vi "MainUI.vi"() -> ()   [LabVIEW 2020]
uses:
  <vilib>/Utility/file.llb/Write Delimited Spreadsheet (string).vi
panel:
  in  "Save flattened data (memory hungry)":bool
  in  "Polarity":T1={"auto detect"=TRUE, "Polarity"=enum."falling"}
  in  "Measurement info":T2={"Det index"=0, "Clk index"=1, "Avg range"=1e-08}
  out "System Waveform Graph":cluster{"t0":dbl, "dt":dbl, "Y":dbl[]}[](graph) caption="ST Screen 3778 w02 no pull 32 - Beam reg23 Setting 7F-7E-7F-7F"
  in  "File extension":string="txt"
  out "Waveform Graph rise":cluster{"t0":dbl, "dt":dbl, "Y":dbl[]}[](graph)
  out "Waveform Graph fall":cluster{"t0":dbl, "dt":dbl, "Y":dbl[]}[](graph)
  out "data":string[](array[string])
  in  "File Path":path
  in  "Save extracted numbers":bool=TRUE
  in  "Filename has to include:":string
  in  "Play":bool
  in  "Exit":bool
  out "Heading":string[](array[string])=["reg23", "State", "Initial", "State", "Final"]
  out "Progress Bar":u8(slide) scale=0.0..100.0
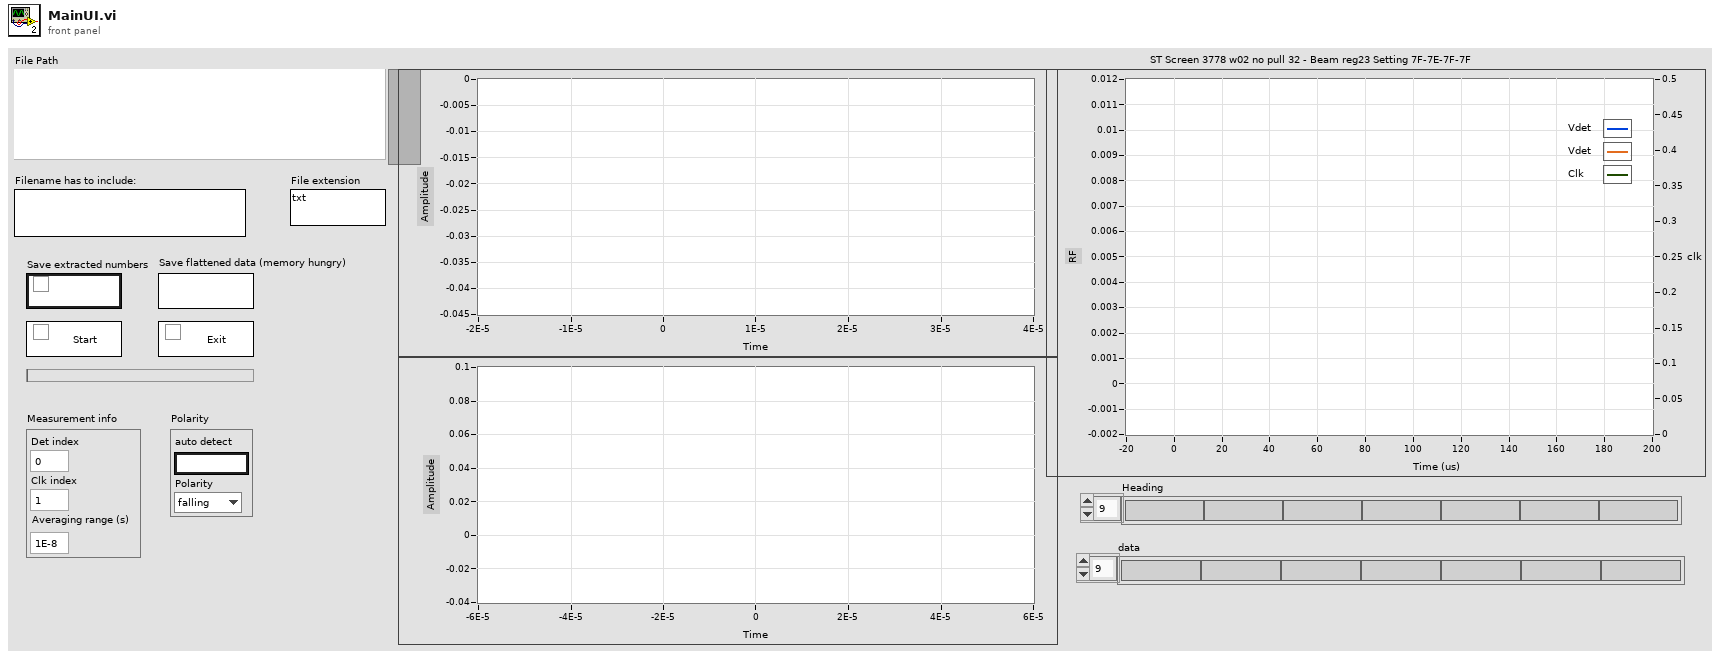
[diagram p1: front panel]
types:
  T1 = cluster{"auto detect":bool, "Polarity":enum16{"falling", "rising"}}
  T2 = cluster{"Det index":i32, "Clk index":i32, "Avg range":dbl}
  T3 = enum8{"Enabled", "Disabled", "Disabled and Grayed Out"}
  T4 = typedef "Timing measurements.ctl" = cluster{"Polarity":enum16{"falling", "rising"}, "low state level":dbl, "high state level":dbl, "t0 (us)":dbl, "Transition duration 10% (us)":dbl, "pre-undershoot 10% (%)":dbl, "pre-overshoot 10% (%)":dbl, "post-undershoot 10% (%)":dbl, "post-overshoot 10% (%)":dbl, "measurement info 10%":cluster{"start time":dbl, "end time":dbl, "ref levels":cluster{"high ref level":dbl, "mid ref level":dbl, "low ref level":dbl, "ref units":u16}}, "Settling time 5% (us)":dbl, "pre-undershoot 5% (%)":dbl, "pre-overshoot 5% (%)":dbl, "post-undershoot 5% (%)":dbl, "post-overshoot 5% (%)":dbl, "measurement info 5%":cluster{"start time":dbl, "end time":dbl, "ref levels":cluster{"high ref level":dbl, "mid ref level":dbl, "low ref level":dbl, "ref units":u16}}, "t0 to 5% (us)":dbl, "t0 to 10% (us)":dbl, "sclk edge":i32}
  T5 = cluster{"start time":dbl, "end time":dbl, "ref levels":cluster{"high ref level":dbl, "mid ref level":dbl, "low ref level":dbl, "ref units":u16}}
  T6 = cluster{"high ref level":dbl, "mid ref level":dbl, "low ref level":dbl, "ref units":u16}
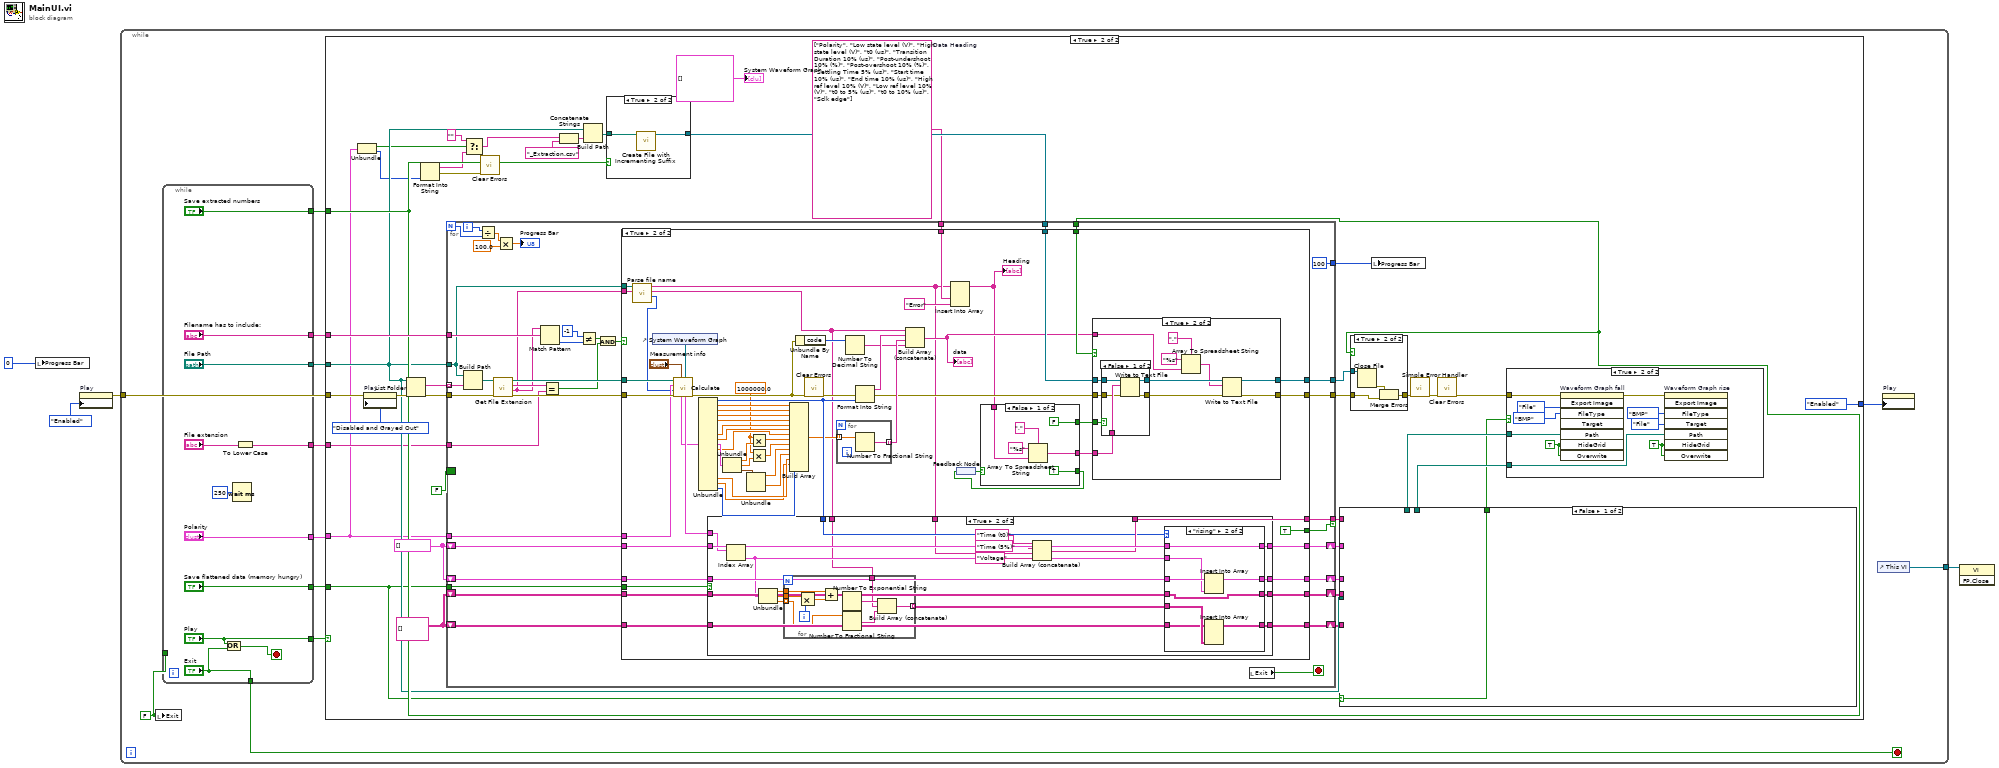
[diagram p0: block diagram]
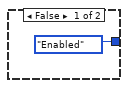
[diagram p2: hidden frame]
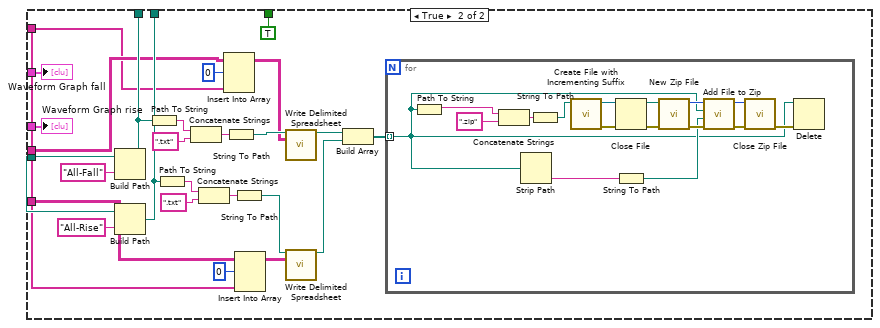
[diagram p4: hidden frame]
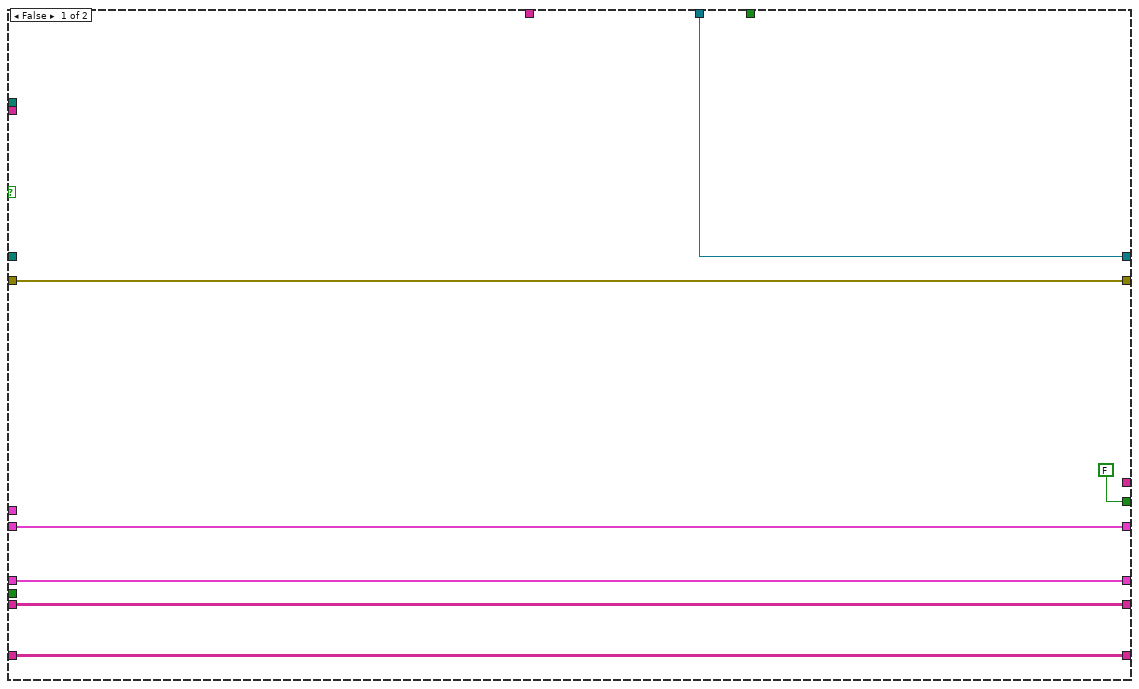
[diagram p7: hidden frame]
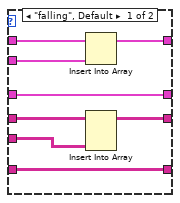
[diagram p9: hidden frame]
diagram:
  n1 = local write "Progress Bar"(u8 0 ("Horizontal Progress Bar")) -> ()
  n2 = property on="Play" class="Bool"("DisabledEnum"=T3."Enabled" ("Disabled")) -> (error out=w2:errorcluster)  [unwired: 2 in, 1 out]
  n3 = while {
    tunnel: w2 -> [w11]
    tunnel: [w8] -> w1
    stop <- w12 stop-if-true
    w10 = FALSE ("Exit")
    n4 = local write "Exit"(w10) -> ()
    n5 = while {
      tunnel: ["File Path"] -> w16
      tunnel: ["Filename has to include:"] -> w15
      tunnel: ["Save extracted numbers"] -> w14
      tunnel: ["Play"] -> w13
      tunnel: ["Exit"] -> w12
      tunnel: w10 -> [_]
      tunnel: [w311] -> w9
      tunnel: ["Polarity"] -> w7
      tunnel: ["Save flattened data (memory hungry)"] -> w5
      stop <- w315 stop-if-true
      n6 = Or(x="Play", y="Exit") -> (x .or. y?=w315:bool)
      n7 = Wait (ms)(milliseconds to wait=u32 250) -> ()  [unwired: 1 out]
      n8 = To Lower Case(string="File extension") -> (all lower case string=w311:string)
    }
    n9 = case shown="True" w13 {
      tunnel: w16 -> [_ w45]
      tunnel: w15 -> [_ w56]
      tunnel: w14 -> [_ w54]
      tunnel: w11 -> [_ w46]
      tunnel: w9 -> [_ w32]
      tunnel: w7 -> [_ w24]
      tunnel: [T3."Enabled" ("Disabled") T3."Enabled" ("Disabled")] -> w6
      tunnel: w5 -> [_ w28]
      frame False {
      }
      frame True {
        w35 = string[] ["Polarity", "Low state level (V)", "High state level (V)", "t0 (us)", "Transition Duration 10% (us)", "Post-undershoot 10% (%)", "Post-overshoot 10% (%)", "Settling Time 5% (us)", "Start time 10% (us)", "End time 10% (us)", "High ref level 10% (V)", "Low ref level 10% (V)", "t0 to 5% (us)", "t0 to 10% (us)", "Sclk edge"]  # Data Heading
        w39 = string[][] []
        w41 = cluster{"t0":dbl, "dt":dbl, "Y":dbl[]}[] []
        n10 = Unbundle(w24) -> ("auto detect"=w23:bool, "Polarity"=w21:enum16{"falling", "rising"})
        n11 = property on="Play" class="Bool"(error in=w46, "DisabledEnum"=T3."Disabled and Grayed Out" ("Disabled")) -> (error out=w48:errorcluster)  [unwired: 1 in, 1 out]
        n12 = List Folder(path=w45, error in=w48) -> (filenames=w58:string[], error out=w57:errorcluster)  [unwired: 2 in, 2 out]
        n13 = Format Into String(w21) -> (resulting string=w20:string, error out=w18:errorcluster)  [unwired: 3 in]
        n14 = Select(t="", s=w23, f=w20) -> (s? t:f=w22:string)
        n15 = call <vilib>:"Clear Errors.vi"("error in (no error)"=w18) -> ()  [unwired: 5 in, 2 out]
        n16 = Concatenate Strings(w22, "_Extraction.csv" ("string")) -> (w25:string)
        n17 = Build Path(base path=w45, name or relative path=w25) -> (appended path=w55:path)
        n18 = case shown="True" w54 {
          tunnel: w55 -> [_ w118]
          tunnel: [_ w117] -> w53
          frame False {
          }
          frame True {
            n19 = call <vilib>:"Create File with Incrementing Suffix.vi"("file path"=w118) -> ("refnum out"=w117:refnum<file>)  [unwired: 8 in, 2 out]
          }
        }
        n20 = for {
          N -> [w146]
          tunnel: w45 -> [w119]
          tunnel: w57 -> [w156]
          tunnel: w58 -> [w123] mode=indexing
          tunnel: w56 -> [w151]
          tunnel: w54 -> [w150]
          tunnel: w53 -> [w149]
          tunnel: [w148] -> w52
          border: FALSE -> [_]
          tunnel: [u8 100 ("Horizontal Progress Bar")] -> w50
          shift-right: [w140] -> w40
          shift-left: w41 -> [w139]
          shift-right: [w137] -> w44
          shift-left: w41 -> [w138]
          shift-right: [w136] -> w38
          shift-left: w39 -> [w134]
          shift-right: [w135] -> w36
          shift-left: w39 -> [w133]
          tunnel: [w132] -> w37 if=w131
          tunnel: w35 -> [w130]
          tunnel: [w129] -> w34
          tunnel: w32 -> [w124]
          tunnel: w24 -> [w122]
          tunnel: w28 -> [w121]
          i -> [w147]
          stop <- w141 stop-if-true
          n21 = Build Path(base path=w119, name or relative path=w123) -> (appended path=w154:path)
          n22 = Divide(x=w147, y=w146) -> (x/y=w145:dbl)
          n23 = call <vilib>:"Get File Extension.vi"("error in (no error)"=w156, "file"=w154) -> ("error out"=w155:errorcluster, "filename without extension"=w120:string, "lowercase file extension"=w126:string, "dup file"=w152:path)  [unwired: 5 in, 1 out]
          n24 = Multiply(x=w145, y=100.0) -> (x*y=→"Progress Bar":dbl)
          n25 = Match Pattern(string=w120, regular expression=w151) -> (offset past match=w153:i32)  [unwired: 1 in, 3 out]
          n26 = Equal?(x=w126, y=w124) -> (x = y?=w125:bool)
          n27 = Not Equal?(x=-1, y=w153) -> (x != y?=w128:bool)
          n28 = And(x=w128, y=w125) -> (x .and. y?=w127:bool)
          n29 = case shown="True" w127 {
            tunnel: w152 -> [_ w218]
            tunnel: [w163 w227] -> w129
            tunnel: w155 -> [w163 w219]
            tunnel: w150 -> [_ w226]
            tunnel: w149 -> [w164 w223]
            tunnel: [w164 w222] -> w148
            tunnel: [w162 w212] -> w140
            tunnel: w139 -> [w162 w213]
            tunnel: w138 -> [w161 w211]
            tunnel: [w161 w210] -> w137
            tunnel: [w159 w209] -> w136
            tunnel: [w160 w208] -> w135
            tunnel: w134 -> [w159 w207]
            tunnel: w133 -> [w160 w206]
            tunnel: [_ w204] -> w132
            tunnel: [FALSE TRUE] -> w131
            tunnel: w130 -> [_ w201]
            tunnel: w122 -> [_ w173]
            tunnel: w121 -> [_ w169]
            tunnel: w120 -> [_ w168]
            tunnel: w119 -> [_ w167]
            frame False {
            }
            frame True {
              w170 = 1000000.0 ("y")
              n30 = call "Parse file name.vi"("filename without extension"=w168, "File Path"=w167) -> ("Changed reg"=w172:u8, "Part info"=w166:string[], "Part info Header"=w165:string[])  [unwired: 7 in]
              n31 = control-ref of="System Waveform Graph"() -> (w180:refnum<vi>)
              n32 = call "Calculate.vi"("WFGraph Refnum"=w180, "Measurement info"="Measurement info", "error in"=w219, "Changed reg"=w172, "Polarity"=w173, "file (use dialog)"=w218) -> ("error out"=w176:errorcluster, "Waveform data out"=w198:cluster{"t0":dbl, "dt":dbl, "Y":dbl[]}[], "Timing measurements"=w197:T4)  [unwired: 1 in, 2 out]
              n33 = Unbundle(w197) -> ("Polarity"=w203:enum16{"falling", "rising"}, "low state level"=w195:dbl, "high state level"=w194:dbl, "t0 (us)"=w193:dbl, "Transition duration 10% (us)"=w192:dbl, "post-undershoot 10% (%)"=w191:dbl, "post-overshoot 10% (%)"=w190:dbl, "measurement info 10%"=w196:T5, "Settling time 5% (us)"=w184:dbl, "t0 to 5% (us)"=w183:dbl, "t0 to 10% (us)"=w182:dbl, "sclk edge"=w171:i32)  [unwired: 7 out]
              n34 = case shown="True" w169 {
                tunnel: w213 -> [w231 w252]
                tunnel: [w231 w251] -> w212
                tunnel: w211 -> [w230 w250]
                tunnel: [w230 w249] -> w210
                tunnel: [w229 w245] -> w209
                tunnel: [w228 w244] -> w208
                tunnel: w207 -> [w229 w243]
                tunnel: w206 -> [w228 w242]
                tunnel: [_ w239] -> w204
                tunnel: w203 -> [_ w237]
                tunnel: w198 -> [_ w236]
                tunnel: w165 -> [_ w233]
                tunnel: w166 -> [_ w232]
                frame False {
                }
                frame True {
                  n35 = Index Array(array=w236) -> (element=w235:cluster{"t0":dbl, "dt":dbl, "Y":dbl[]})  [unwired: 1 in]
                  n36 = Unbundle(w235) -> ("t0"=w247:dbl, "dt"=w246:dbl, "Y"=w248:dbl[])
                  n37 = for {
                    tunnel: w248 -> [w259] mode=indexing
                    tunnel: w247 -> [w260]
                    tunnel: w246 -> [w261]
                    tunnel: w232 -> [w257]
                    tunnel: [w255] -> w238 mode=indexing
                    i -> [w262]
                    n38 = Multiply(x=w261, y=w262) -> (x*y=w253:dbl)
                    n39 = Add(x=w260, y=w253) -> (x+y=w254:dbl)
                    n40 = Number To Exponential String(number=w254) -> (E-format string=w258:string)  [unwired: 3 in]
                    n41 = Number To Fractional String(number=w259) -> (F-format string=w256:string)  [unwired: 3 in]
                    n42 = Build Array (concatenate)(w258, w257, w256) -> (w255:string[])
                  }
                  n43 = Build Array (concatenate)("Time (t0)", "Time (5%)", w233, "Voltage") -> (w239:string[])
                  n44 = case shown="\"rising\"" w237 {
                    tunnel: w235 -> [w270 w275]
                    tunnel: w252 -> [w269 w278]
                    tunnel: [w268 w278] -> w251
                    tunnel: w250 -> [w267 w277]
                    tunnel: [w267 w276] -> w249
                    tunnel: [w266 w271] -> w245
                    tunnel: w238 -> [w265 w274]
                    tunnel: [w263 w273] -> w244
                    tunnel: w243 -> [w264 w271]
                    tunnel: w242 -> [w263 w272]
                    frame "falling", Default {
                      n45 = Insert Into Array(array=w269, new element=w270) -> (w268:cluster{"t0":dbl, "dt":dbl, "Y":dbl[]}[])  [unwired: 1 in]
                      n46 = Insert Into Array(array=w264, new element=w265) -> (w266:string[][])  [unwired: 2 in]
                    }
                    frame "rising" {
                      n47 = Insert Into Array(array=w277, new element=w275) -> (w276:cluster{"t0":dbl, "dt":dbl, "Y":dbl[]}[])  [unwired: 1 in]
                      n48 = Insert Into Array(array=w272, new element=w274) -> (w273:string[][])  [unwired: 2 in]
                    }
                  }
                }
              }
              n49 = Unbundle(w196) -> ("start time"=w200:dbl, "end time"=w199:dbl, "ref levels"=w202:T6)
              n50 = Unbundle(w202) -> ("high ref level"=w187:dbl, "low ref level"=w186:dbl)  [unwired: 2 out]
              n51 = Multiply(x=w170, y=w200) -> (x*y=w189:dbl)
              n52 = Multiply(x=w170, y=w199) -> (x*y=w188:dbl)
              n53 = Build Array(w195, w194, w193, w192, w191, w190, w184, w189, w188, w187, w186, w183, w182, w171) -> (w185:dbl[])
              n54 = Unbundle By Name(w176) -> ("code"=w175:i32)
              n55 = call <vilib>:"Clear Errors.vi"("error in (no error)"=w176) -> ("error out"=w177:errorcluster)  [unwired: 5 in, 1 out]
              n56 = for {
                tunnel: [w280] -> w217 mode=indexing
                tunnel: w185 -> [w279] mode=indexing
                n57 = Number To Fractional String(number=w279) -> (F-format string=w280:string)  [unwired: 3 in]
              }
              n58 = Number To Decimal String(number=w175) -> (decimal integer string=w174:string)  [unwired: 1 in]
              n59 = Format Into String(error in=w177, w203) -> (resulting string=w215:string, error out=w216:errorcluster)  [unwired: 2 in]
              n60 = Build Array (concatenate)(w166, w215, w217, w174) -> (w214:string[])
              "data" <- w214
              n61 = Insert Into Array(array=w165, new element #1=w201, new element #2="Error" ("new element/subarray")) -> (w179:string[])  [unwired: 1 in]
              "Heading" <- w179
              n62 = feedback #1() -> (w221:bool)
              n63 = case shown="False" w221 {
                selector: w221 -> [_ w287]
                tunnel: [TRUE w287] -> w220
                tunnel: [w283 _] -> w225
                tunnel: [FALSE w287] -> w224
                tunnel: w179 -> [w281 _]
                frame False {
                  n64 = Array To Spreadsheet String(delimiter (Tab)=",", array=w281, 3:"%s" ("format string")) -> (spreadsheet string=w283:string)
                }
                frame True {
                }
              }
              n65 = feedback-in #1(w220) -> ()
              n66 = case shown="True" w226 {
                tunnel: [w288 w301] -> w227
                tunnel: w225 -> [_ w300]
                tunnel: w224 -> [_ w297]
                tunnel: w223 -> [w289 w295]
                tunnel: [w289 w296] -> w222
                tunnel: w214 -> [_ w294]
                tunnel: w216 -> [w288 w293]
                frame False {
                }
                frame True {
                  n67 = case shown="False" w297 {
                    tunnel: w300 -> [w306 _]
                    tunnel: [w305 w307] -> w299
                    tunnel: [w303 w308] -> w298
                    tunnel: w295 -> [w304 w308]
                    tunnel: w293 -> [w302 w307]
                    frame False {
                      n68 = Write to Text File(file (use dialog)=w304, text=w306, error in=w302) -> (refnum out=w303:refnum<file>, error out=w305:errorcluster)  [unwired: 1 in, 1 out]
                    }
                    frame True {
                    }
                  }
                  n69 = Array To Spreadsheet String(delimiter (Tab)=",", array=w294, 3:"%s" ("format string")) -> (spreadsheet string=w290:string)
                  n70 = Write to Text File(file (use dialog)=w298, text=w290, error in=w299) -> (refnum out=w296:refnum<file>, error out=w301:errorcluster)  [unwired: 1 in, 1 out]
                }
              }
            }
          }
          n71 = local read "Exit"() -> (w141:bool)
        }
        n72 = case shown="False" w28 {
          selector: w28 -> [w69 _]
          tunnel: w45 -> [_ w93]
          tunnel: w44 -> [_ w92]
          tunnel: [_ w89] -> w43
          tunnel: [_ w85] -> w42
          tunnel: w40 -> [_ w83]
          tunnel: w38 -> [_ w80]
          tunnel: w37 -> [_ w76]
          tunnel: w36 -> [_ w75]
          tunnel: [w69 TRUE] -> w27
          frame False {
          }
          frame True {
            n73 = Build Path(base path=w93, name or relative path="All-Fall") -> (appended path=w89:path)
            n74 = Build Path(base path=w93, name or relative path="All-Rise") -> (appended path=w85:path)
            n75 = Path To String(path=w89) -> (string=w84:string)
            n76 = Path To String(path=w85) -> (string=w87:string)
            n77 = Concatenate Strings(w84, ".txt" ("format string")) -> (w90:string)
            n78 = Concatenate Strings(w87, ".txt" ("format string")) -> (w88:string)
            n79 = Insert Into Array(array=w80, index (row)=0, new element=w76) -> (w78:string[][])  [unwired: 1 in]
            n80 = String To Path(string=w90) -> (path=w82:path)
            n81 = String To Path(string=w88) -> (path=w81:path)
            n82 = Insert Into Array(array=w75, index (row)=0, new element=w76) -> (w74:string[][])  [unwired: 1 in]
            n83 = call-poly <vilib>:"Write Delimited Spreadsheet.vi"("file path (dialog if empty)"=w82, "2D data"=w78) -> ("new file path (Not A Path if cancelled)"=w73:path)  [unwired: 12 in, 1 out]
            n84 = call-poly <vilib>:"Write Delimited Spreadsheet.vi"("file path (dialog if empty)"=w81, "2D data"=w74) -> ("new file path (Not A Path if cancelled)"=w71:path)  [unwired: 12 in, 1 out]
            n85 = Build Array(w73, w71) -> (w72:path[])
            n86 = for {
              tunnel: w72 -> [w96] mode=indexing
              n87 = Path To String(path=w96) -> (string=w99:string)
              n88 = Concatenate Strings(w99, ".zip" ("name or relative path")) -> (w110:string)
              n89 = Strip Path(path=w96) -> (name=w98:string)  [unwired: 1 out]
              n90 = String To Path(string=w110) -> (path=w102:path)
              n91 = call <vilib>:"Create File with Incrementing Suffix.vi"("file path"=w102) -> ("error out"=w103:errorcluster, "refnum out"=w104:refnum<file>)  [unwired: 8 in, 1 out]
              n92 = Close File(refnum=w104, error in=w103) -> (path=w101:path, error out=w100:errorcluster)
              n93 = String To Path(string=w98) -> (path=w97:path)
              n94 = call <vilib>:"New Zip File.vi"("error in (no error)"=w100, "target"=w101) -> ("error out"=w109:errorcluster, "zip file out"=w108:i64)  [unwired: 3 in, 1 out]
              n95 = call <vilib>:"Add File to Zip.vi"("error in (no error)"=w109, "destination path in zip"=w97, "source file path"=w96, "zip file in"=w108) -> ("error out"=w106:errorcluster, "zip file out"=w107:i64)  [unwired: 6 in]
              n96 = call <vilib>:"Close Zip File.vi"("error in (no error)"=w106, "zip file in"=w107) -> ("error out"=w105:errorcluster)  [unwired: 5 in]
              n97 = Delete(path (use dialog)=w96, error in=w105) -> ()  [unwired: 3 in, 3 out]
            }
            "Waveform Graph fall" <- w83
            "Waveform Graph rise" <- w92
          }
        }
        n98 = case shown="True" w54 {
          tunnel: w52 -> [_ w116]
          tunnel: w34 -> [w112 w114]
          tunnel: [w112 w113] -> w33
          frame False {
          }
          frame True {
            n99 = Close File(refnum=w116) -> (error out=w115:errorcluster)  [unwired: 1 in, 1 out]
            n100 = Merge Errors(w115, w114) -> (w113:errorcluster)
          }
        }
        n101 = local write "Progress Bar"(w50) -> ()
        n102 = call <vilib>:"Simple Error Handler.vi"("error in (no error)"=w33) -> ("error out"=w47:errorcluster)  [unwired: 4 in, 4 out]
        n103 = call <vilib>:"Clear Errors.vi"("error in (no error)"=w47) -> ("error out"=w30:errorcluster)  [unwired: 5 in, 1 out]
        n104 = case shown="True" w27 {
          tunnel: w43 -> [_ w61]
          tunnel: w42 -> [_ w60]
          tunnel: w30 -> [_ w59]
          frame False {
          }
          frame True {
            w62 = TRUE ("Hide Grid")
            w63 = TRUE ("Hide Grid")
            n105 = invoke on="Waveform Graph fall" class="WFGraph (strict)" method="Export Image"(error in=w59, "FileType"=enum32{"BMP", "EPS", "EMF", "PICT"}."BMP" ("File Type"), "Target"=enum32{"File", "Clipboard"}."File", "Path"=w61, "HideGrid"=w63, "Overwrite"=w63) -> (error out=w66:errorcluster)  [unwired: 2 in, 7 out]
            n106 = invoke on="Waveform Graph rise" class="WFGraph (strict)" method="Export Image"(error in=w66, "FileType"=enum32{"BMP", "EPS", "EMF", "PICT"}."BMP" ("File Type"), "Target"=enum32{"File", "Clipboard"}."File", "Path"=w60, "HideGrid"=w62, "Overwrite"=w62) -> ()  [unwired: 2 in, 8 out]
          }
        }
        "System Waveform Graph" <- cluster{"t0":dbl, "dt":dbl, "Y":dbl[]}[] []
      }
    }
    n107 = control-ref of="This VI"() -> (w8:refnum<vi>)
    n108 = property on="Play" class="Bool"("DisabledEnum"=w6) -> ()  [unwired: 2 in, 2 out]
  }
  n109 = invoke class="VI" method="FP.Close"(reference=w1) -> ()  [unwired: 2 in, 3 out]
